vi "Connection to String.vi"(8 "error in (no error)":errorcluster, 9 "Create module property if it doesn't exist? (T)":bool=TRUE, 10 "Connection":T2, 11 "Routing and Faulting Ref in":T1 format="%.0x") -> (0 "error out":errorcluster, 1 "Conversion successful?":bool, 2 "String":string, 3 "Routing and Faulting Ref out":T1 format="%.0x")   [LabVIEW 2017, in "Routing and Faulting Scripting.lvlib"]
uses:
  Routing and Faulting Scripting.lvlib
  Shared/Connection.ctl
  <vilib>/NI Veristand/Custom Device API/Custom Device Item Ref.ctl
  NationalInstruments.VeriStand.SystemDefinitionAPI
  NationalInstruments.VeriStand.SystemStorage
  Constants/Scripting Constants.vi
  Shared/Routing and Faulting Shared.lvlib
  <vilib>/NI Veristand/Custom Device API/Custom Device API.lvlib
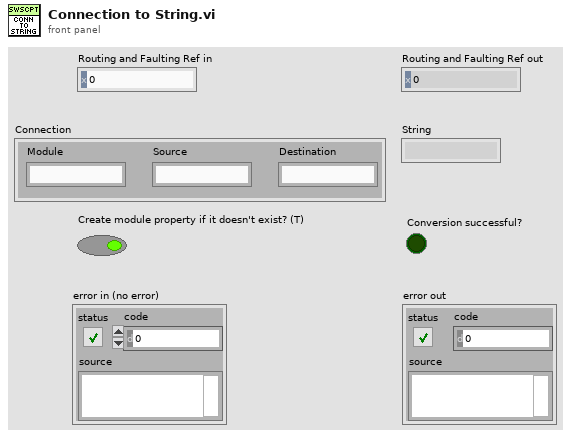
[diagram p1: front panel]
types:
  T1 = typedef "Custom Device API.lvlib/Custom Device Item Ref.ctl" = u64
  T2 = typedef "Routing and Faulting Shared.lvlib/Connection.ctl" = cluster{"Module":string, "Source":string, "Destination":string}
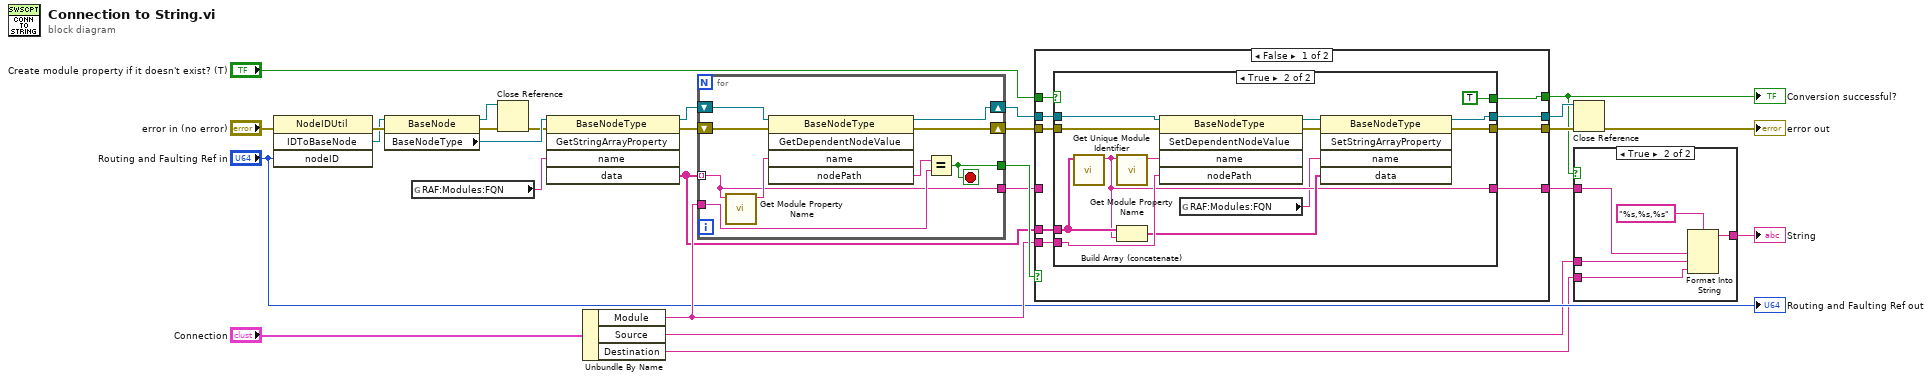
[diagram p0: block diagram]
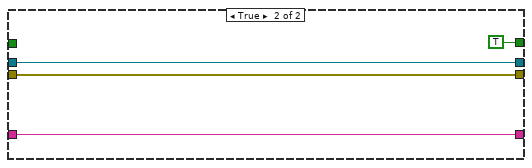
[diagram p4: hidden frame]
diagram:
  n1 = invoke class="NodeIDUtil" method="IDToBaseNode"(error in="error in (no error)", "nodeID"="Routing and Faulting Ref in") -> (error out=w26:errorcluster, "IDToBaseNode"=w25:refnum<k24>)  [unwired: 2 in, 2 out]
  n2 = property class="BaseNode"(reference=w25, error in=w26) -> (reference out=w10:refnum<k24>, error out=w14:errorcluster, "BaseNodeType"=w15:refnum<k24>)
  n3 = global read "Scripting Constants.vi" "RAF:Modules:FQN"() -> (w7:string)
  n4 = Close Reference(reference=w10, error in (no error)=w14) -> (error out=w11:errorcluster)
  n5 = invoke class="BaseNodeType" method="GetStringArrayProperty"(reference=w15, error in=w11, "name"=w7) -> (reference out=w23:refnum<k24>, error out=w24:errorcluster, "data"=w17:string[])  [unwired: 2 in, 2 out]
  n6 = Unbundle By Name("Connection") -> ("Module"=w18:string, "Source"=w6:string, "Destination"=w5:string)
  n7 = for {
    tunnel: w17 -> [w28] mode=indexing
    tunnel: w18 -> [w29]
    tunnel: [w28] -> w16
    shift-right: [w33] -> w21
    shift-left: w24 -> [w36]
    tunnel: [w32] -> w22
    shift-right: [w31] -> w19
    shift-left: w23 -> [w35]
    stop <- w32 stop-if-true
    n8 = call "Get Module Property Name.vi"("Module ID"=w28) -> ("Module Property Name"=w30:string)  [unwired: 10 in]
    n9 = invoke class="BaseNodeType" method="GetDependentNodeValue"(reference=w35, error in=w36, "name"=w30) -> (reference out=w31:refnum<k24>, error out=w33:errorcluster, "nodePath"=w34:string)  [unwired: 2 in, 2 out]
    n10 = Equal?(x=w34, y=w29) -> (x = y?=w32:bool)
  }
  n11 = case shown="False" w22 {
    tunnel: w21 -> [w45 w64]
    tunnel: [w42 w64] -> w20
    tunnel: w19 -> [w44 w62]
    tunnel: w18 -> [w43 _]
    tunnel: w17 -> [w41 _]
    tunnel: w16 -> [_ w63]
    tunnel: [w40 w63] -> w3
    tunnel: [w39 w62] -> w8
    tunnel: "Create module property if it doesn't exist? (T)" -> [w38 _]
    tunnel: [w37 TRUE] -> w1
    frame False {
      n12 = case shown="True" w38 {
        tunnel: w45 -> [w47 w60]
        tunnel: w44 -> [w46 w59]
        tunnel: w43 -> [_ w58]
        tunnel: [w47 w55] -> w42
        tunnel: w41 -> [_ w53]
        tunnel: [_ w51] -> w40
        tunnel: [w46 w50] -> w39
        tunnel: [_ TRUE] -> w37
        frame False {
        }
        frame True {
          n13 = call "Get Unique Module Identifier.vi"("Existing Module Identifiers"=w53) -> ("Unique Module Identifier"=w51:string)  [unwired: 10 in]
          n14 = call "Get Module Property Name.vi"("Module ID"=w51) -> ("Module Property Name"=w57:string)  [unwired: 10 in]
          n15 = Build Array (concatenate)(w53, w51) -> (w52:string[])
          n16 = invoke class="BaseNodeType" method="SetDependentNodeValue"(reference=w59, error in=w60, "name"=w57, "nodePath"=w58) -> (reference out=w56:refnum<k24>, error out=w54:errorcluster)  [unwired: 1 in, 3 out]
          n17 = global read "Scripting Constants.vi" "RAF:Modules:FQN"() -> (w49:string)
          n18 = invoke class="BaseNodeType" method="SetStringArrayProperty"(reference=w56, error in=w54, "name"=w49, "data"=w52) -> (reference out=w50:refnum<k24>, error out=w55:errorcluster)  [unwired: 1 in, 3 out]
        }
      }
    }
    frame True {
    }
  }
  "Conversion successful?" <- w1
  n19 = Close Reference(reference=w8, error in (no error)=w20) -> (error out=→"error out":errorcluster)
  n20 = case shown="True" w1 {
    tunnel: w6 -> [_ w69]
    tunnel: w5 -> [_ w68]
    tunnel: [_ w67] -> w4
    tunnel: w3 -> [_ w65]
    frame False {
    }
    frame True {
      n21 = Format Into String(format string="%s,%s,%s", w65, w69, w68) -> (resulting string=w67:string)  [unwired: 2 in, 1 out]
    }
  }
  "String" <- w4
  "Routing and Faulting Ref out" <- "Routing and Faulting Ref in"
